vi "OAT Truncate Time Indices.vi"(6 "last indices":dbl format="%.2f", 7 "reset? (True)":bool=TRUE, 8 "spectral settings":T2={"window type"=1, "number of lines"=400} {"number of lines" min=2; "window type" items=["None"=0, "Hanning"=1, "Hamming"=2, "Blackman-Harris"=3, "Exact Blackman"=4, "Blackman"=5, "Flat Top"=6, "4 Term B-Harris"=7, "7 Term B-Harris"=8, "Low Sidelobe"=9, "Gaussian"=62]}, 9 "X scale in":cluster{"offset":dbl, "multiplier":dbl} {"multiplier" format="%.2f"; "offset" format="%.2f"}, 10 "time in":dbl[](array[numeric])=[17.400000000000002, 17.6] format="%.2f", 11 "scaled signal [EU] in":waveform(dbl)) -> (0 "finished":bool, 1 "scales":T1 {"Y scale"."multiplier" format="%.2f"; "Y scale"."offset" format="%.2f"; "X scale"."multiplier" format="%.2f"; "X scale"."offset" format="%.2f"}, 2 "window indices":dbl[](array[numeric]), 3 "data out":dbl[](array[numeric]) format="%.2f")   [LabVIEW 2017, in "SoundVib_Resampling.lvlib"]
uses:
  <vilib>/addons/Sound and Vibration/Order Analysis/Resample Order Tracking/SoundVib_Resampling.lvlib
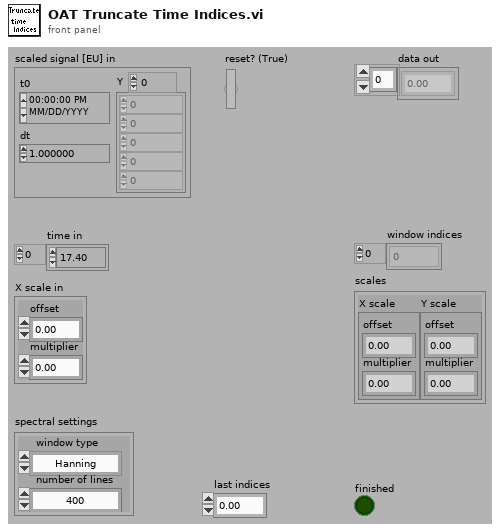
[diagram p1: front panel]
types:
  T1 = cluster{"X scale":cluster{"offset":dbl, "multiplier":dbl}, "Y scale":cluster{"offset":dbl, "multiplier":dbl}}
  T2 = cluster{"window type":u32, "number of lines":i32}
  T3 = cluster{"X scale in":cluster{"offset":dbl, "multiplier":dbl}, cluster{"x/y":dbl, dbl}}
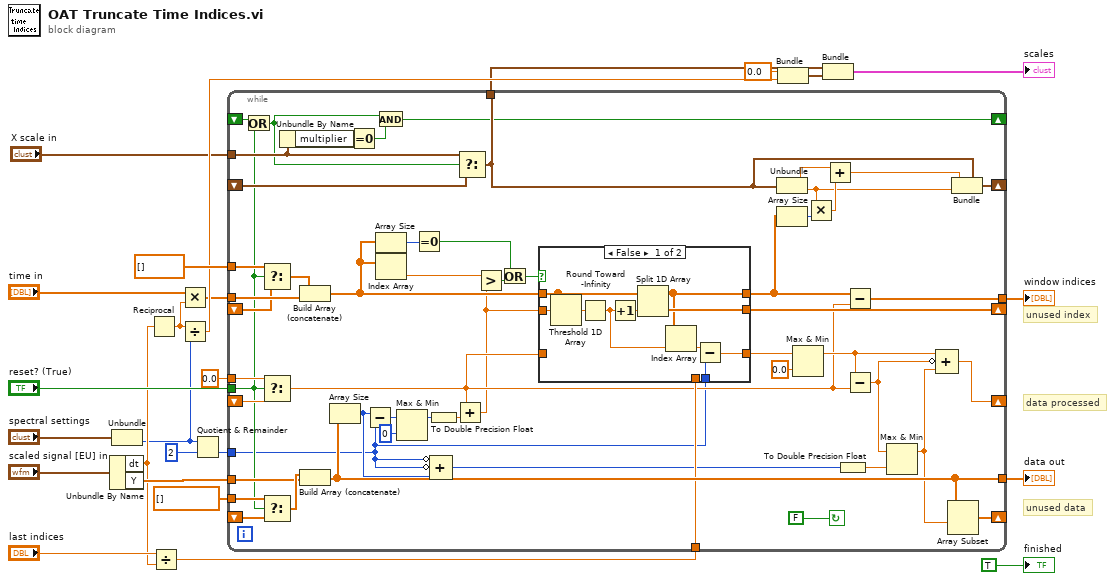
[diagram p0: block diagram]
diagram:
  # "unused data"
  # "unused index"
  # "data processed"
  n1 = Unbundle By Name("scaled signal [EU] in") -> ("dt"=w7:dbl, "Y"=w20:dbl[])
  n2 = Unbundle("spectral settings") -> ("number of lines"=w6:i32)  [unwired: 1 out]
  n3 = Reciprocal(x=w7) -> (1/x=w13:dbl)
  n4 = Divide(x="last indices", y=w7) -> (x/y=w3:dbl)
  n5 = Multiply(x="time in", y=w13) -> (x*y=w4:dbl[])
  n6 = Divide(x=w13, y=w6) -> (x/y=w12:dbl)
  n7 = Quotient & Remainder(x=w6, y=2) -> (floor(x/y)=w5:i32)  [unwired: 1 out]
  n8 = while {
    shift-right: [w76] -> _
    shift-left: _ -> [w72]
    tunnel: w20 -> [w65]
    shift-right: [w28] -> _
    shift-left: _ -> [w77]
    tunnel: w4 -> [w75]
    tunnel: 0.0 -> [w79]
    shift-right: [w70] -> _
    shift-left: _ -> [w73]
    tunnel: "reset? (True)" -> [w43]
    tunnel: [w69] -> w21
    tunnel: dbl[] [] ("t") -> [w74]
    tunnel: dbl[] [] ("t") -> [w71]
    tunnel: [w64] -> w15
    tunnel: w5 -> [w31]
    tunnel: w3 -> [w55]
    shift-right: [w56] -> _
    shift-left: _ -> [w51]
    tunnel: "X scale in" -> [w48]
    tunnel: [w49] -> w2
    shift-right: [w41] -> _
    shift-left: _ -> [w44]
    stop <- FALSE continue-if-true
    n9 = Or(x=w44, y=w43) -> (x .or. y?=w42:bool)
    n10 = Select(t=w74, s=w43, f=w73) -> (s? t:f=w61:dbl[])
    n11 = Select(t=w79, s=w43, f=w77) -> (s? t:f=w39:dbl)
    n12 = Select(t=w71, s=w43, f=w72) -> (s? t:f=w66:dbl[])
    n13 = Unbundle By Name(w48) -> ("multiplier"=w46:dbl)
    n14 = Build Array (concatenate)(w61, w75) -> (w38:dbl[])
    n15 = Build Array (concatenate)(w66, w65) -> (w64:dbl[])
    n16 = Array Size(array=w64) -> (size(s)=w32:i32)
    n17 = Equal To 0?(x=w46) -> (x = 0?=w45:bool)
    n18 = Subtract(x=w32, y=w31) -> (x-y=w67:i32)
    n19 = And(x=w42, y=w45) -> (x .and. y?=w41:bool)
    n20 = Array Size(array=w38) -> (size(s)=w68:i32)
    n21 = Index Array(array=w38) -> (element=w37:dbl)  [unwired: 1 in]
    n22 = Max & Min(x=w67, y=0) -> (max(x,y)=w63:i32)  [unwired: 1 out]
    n23 = Equal To 0?(x=w68) -> (x = 0?=w34:bool)
    n24 = To Double Precision Float(number=w63) -> (double precision float=w52:dbl)
    n25 = Compound Arithmetic op=ADD(invert w31, invert w31, w32) -> (w30:i32)
    n26 = Add(x=w39, y=w52) -> (x+y=w36:dbl)
    n27 = Select(t=w48, s=w42, f=w51) -> (s? t:f=w49:cluster{"offset":dbl, "multiplier":dbl})
    n28 = Greater?(x=w37, y=w36) -> (0:w35:bool)
    n29 = Or(x=w34, y=w35) -> (x .or. y?=w33:bool)
    n30 = case shown="False" w33 {
      tunnel: w36 -> [w89 _]
      tunnel: [w88 w91] -> w70
      tunnel: w38 -> [w87 w91]
      tunnel: w55 -> [_ _]
      tunnel: [w86 _] -> w50
      tunnel: [w84 w90] -> w40
      tunnel: w31 -> [w83 _]
      tunnel: w39 -> [_ w90]
      frame False {
        n31 = Threshold 1D Array(2:w89, 3:w87) -> (0:w85:dbl)  [unwired: 1 in]
        n32 = Round Toward -Infinity(1:w85) -> (0:w82:dbl)
        n33 = Increment(x=w82) -> (x+1=w81:dbl)
        n34 = Split 1D Array(array=w87, index=w81) -> (first subarray=w86:dbl[], second subarray=w88:dbl[])
        n35 = Index Array(array=w86, index=w82) -> (element=w80:dbl)
        n36 = Subtract(x=w80, y=w83) -> (x-y=w84:dbl)
      }
      frame True {
      }
    }
    n37 = Unbundle(w49) -> ("offset"=w58:dbl, "multiplier"=w47:dbl)
    n38 = Array Size(array=w50) -> (size(s)=w60:i32)
    n39 = Max & Min(x=w40, y=0.0) -> (max(x,y)=w53:dbl)  [unwired: 1 out]
    n40 = Multiply(x=w47, y=w60) -> (x*y=w59:dbl)
    n41 = Add(x=w58, y=w59) -> (x+y=w57:dbl)
    n42 = To Double Precision Float(number=w30) -> (double precision float=w29:dbl)
    n43 = Subtract(x=w50, y=w39) -> (x-y=w69:dbl[])
    n44 = Subtract(x=w53, y=w39) -> (x-y=w27:dbl)
    n45 = Max & Min(x=w27, y=w29) -> (max(x,y)=w26:dbl)  [unwired: 1 out]
    n46 = Compound Arithmetic op=ADD(w53, invert w27, w26) -> (w28:dbl)
    n47 = Array Subset(array=w64, index=w26) -> (w76:dbl[])  [unwired: 1 in]
    n48 = Bundle(cluster=w49, "offset"=w57, "multiplier"=w47) -> (w56:cluster{"offset":dbl, "multiplier":dbl})
  }
  "data out" <- w15
  "window indices" <- w21
  n49 = Bundle("x/y"=0.0, w12) -> (w10:cluster{"x/y":dbl, dbl})  [unwired: 1 in]
  n50 = Bundle("X scale in"=w2, w10) -> (→"scales":T3)  [unwired: 1 in]
  "finished" <- TRUE ("finished")
